vi "WriteClock.vi"(6 "Error In":errorcluster, 7 "Time & Date":u8[](array[numeric])=[0], 8 "Cluster":T1, 9 "LINX Resource":T2={"IO"=enum."Remote", "Interface"=enum."Serial", "LINX Device Config"={"Interface"=enum."Serial", "COM Port"="COM13", "TCP Configuration"={"IP Address"="", "Port"=0}, "Device Family"=1, "Device ID"=1, "Device Name"="myRIO-1900", "TCP Ref"=refnum, "Channels"={"DI"=[0, 1, 2, 3, 4, 5, 6, 7, 8, 9, 10, 11, 12, 13, 14, 15, 16, 17, 18, 19, 20, 21, 22, 23, 24, 25, 26, 27, 28, 29, 30, 31, 32, 33, 34, 35, 36, 37, 38, 39, 40, 41, 42, 43, 44, 45, 46], "DO"=[0, 1, 2, 3, 4, 5, 6, 7, 8, 9, 10, 11, 12, 13, 14, 15, 16, 17, 18, 19, 20, 21, 22, 23, 24, 25, 26, 27, 28, 29, 30, 31, 32, 33, 34, 35, 36, 37, 38, 39, 40, 41, 42, 43, 44, 45, 46], "AI"=[0, 1, 2, 3, 4, 5, 6, 7, 8, 9, 10, 11], "AO"=[], "PWM"=[3, 5, 6, 9, 10], "QE"=[], "UART"=[0, 1], "I2C 2"=[0], "SPI"=[0], "CAN"=[], "Servo"=[], "AI Ref (V)"=0.0, "AI Resolution (Bits)"=0, "AO Ref (V)"=0.0, "AO Resolution (Bits)"=0}}}) -> (0 "Error Out":errorcluster, 3 "LINX Resource":T2={"IO"=enum."Remote", "Interface"=enum."Serial", "LINX Device Config"={"Interface"=enum."Serial", "COM Port"="COM13", "TCP Configuration"={"IP Address"="", "Port"=0}, "Device Family"=1, "Device ID"=1, "Device Name"="myRIO-1900", "TCP Ref"=refnum, "Channels"={"DI"=[0, 1, 2, 3, 4, 5, 6, 7, 8, 9, 10, 11, 12, 13, 14, 15, 16, 17, 18, 19, 20, 21, 22, 23, 24, 25, 26, 27, 28, 29, 30, 31, 32, 33, 34, 35, 36, 37, 38, 39, 40, 41, 42, 43, 44, 45, 46], "DO"=[0, 1, 2, 3, 4, 5, 6, 7, 8, 9, 10, 11, 12, 13, 14, 15, 16, 17, 18, 19, 20, 21, 22, 23, 24, 25, 26, 27, 28, 29, 30, 31, 32, 33, 34, 35, 36, 37, 38, 39, 40, 41, 42, 43, 44, 45, 46], "AI"=[0, 1, 2, 3, 4, 5, 6, 7, 8, 9, 10, 11], "AO"=[], "PWM"=[3, 5, 6, 9, 10], "QE"=[], "UART"=[0, 1], "I2C 2"=[0], "SPI"=[0], "CAN"=[], "Servo"=[], "AI Ref (V)"=0.0, "AI Resolution (Bits)"=0, "AO Ref (V)"=0.0, "AO Resolution (Bits)"=0}}})   [LabVIEW 2024]
uses:
  <vilib>/MakerHub/LINX/Private/Type Defs/LINX Ref.ctl
  <vilib>/MakerHub/LINX/Private/Type Defs/Platform.ctl
  <vilib>/MakerHub/LINX/Private/Type Defs/Interface.ctl
  <vilib>/MakerHub/LINX/Private/Device/Type Defs/LINX Device Config.ctl
  <vilib>/MakerHub/LINX/Private/Device/Type Defs/TCP Config.ctl
  <vilib>/MakerHub/LINX/Private/Device/Type Defs/Channels.ctl
  <vilib>/MakerHub/LINX/Private/Local IO/LinxI2cWrite.vi
  <vilib>/MakerHub/LINX/Public/Utilities/Check Channel.vi
  <vilib>/MakerHub/LINX/Private/Local IO/Handle Errors.vi
  <vilib>/MakerHub/LINX/Private/Utilties/Generate Error.vi
  <vilib>/MakerHub/LINX/LMH-LINX.lvlib
  <vilib>/MakerHub/LINX/Private/Device/Device.lvlib
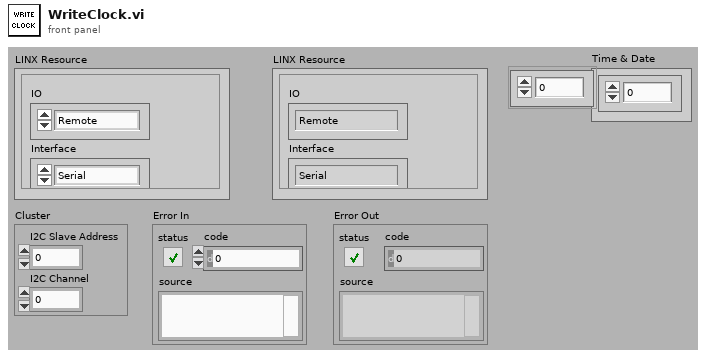
[diagram p1: front panel]
types:
  T1 = cluster{"I2C Slave Address":u8, "I2C Channel":u8}
  T2 = typedef "LMH-LINX.lvlib/LINX Ref.ctl" = cluster{"IO":T3, "Interface":T4, "LINX Device Config":T5}
  T3 = typedef "LMH-LINX.lvlib/Platform.ctl" = enum16{"Remote", "Local"}
  T4 = typedef "LMH-LINX.lvlib/Interface.ctl" = enum16{"Serial", "TCP"}
  T5 = typedef "LMH-LINX.lvlib/Device.lvlib/LINX Device Config.ctl" = cluster{"Interface":T4, "COM Port":refnum<visa-resource-name>, "TCP Configuration":T6, "Device Family":u8, "Device ID":u8, "Device Name":string, "TCP Ref":refnum<k5>, "Channels":T7}
  T6 = typedef "LMH-LINX.lvlib/Device.lvlib/TCP Config.ctl" = cluster{"IP Address":string, "Port":u16}
  T7 = typedef "LMH-LINX.lvlib/Channels.ctl" = cluster{"DI":u8[], "DO":u8[], "AI":u8[], "AO":u8[], "PWM":u8[], "QE":u8[], "UART":u8[], "I2C 2":u8[], "SPI":u8[], "CAN":u8[], "Servo":u8[], "AI Ref (V)":dbl, "AI Resolution (Bits)":u8, "AO Ref (V)":dbl, "AO Resolution (Bits)":u8}
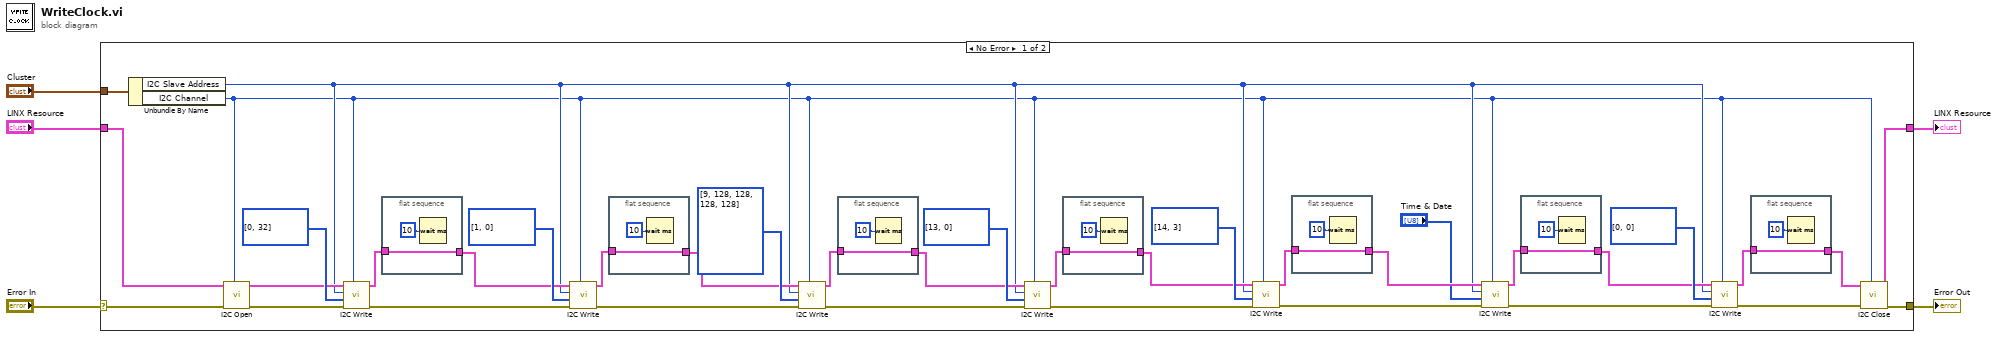
[diagram p0: block diagram]
diagram:
  n1 = case shown="No Error" "Error In" {
    selector: "Error In" -> [w35 w58]
    tunnel: [w41 w58] -> w3
    tunnel: "LINX Resource" -> [w42 w57]
    tunnel: [w40 w57] -> w4
    tunnel: "Cluster" -> [w34 _]
    frame No Error {
      n2 = Unbundle By Name(w34) -> ("I2C Slave Address"=w8:u8, "I2C Channel"=w7:u8)
      n3 = call <vilib>:"I2C Open.vi"("I2C Channel (0)"=w7, "Error In"=w35, "LINX Resource"=w42) -> ("Error Out"=w36:errorcluster, "LINX Resource"=w38:T2)  [unwired: 7 in]
      n4 = call <vilib>:"I2C Write.vi"("I2C Channel"=w7, "Error In"=w36, "Data"=u8[] [0, 32], "I2C Slave Address (0)"=w8, "LINX Resource"=w38) -> ("Error Out"=w26:errorcluster, "LINX Resource"=w37:T2)  [unwired: 5 in]
      n5 = flat-sequence {
        tunnel: [w56] -> w27
        tunnel: w37 -> [w56]
        frame #0 {
          n6 = Wait (ms)(milliseconds to wait=u32 10) -> ()  [unwired: 1 out]
        }
      }
      n7 = call <vilib>:"I2C Write.vi"("I2C Channel"=w7, "Error In"=w26, "Data"=u8[] [1, 0], "I2C Slave Address (0)"=w8, "LINX Resource"=w27) -> ("Error Out"=w25:errorcluster, "LINX Resource"=w33:T2)  [unwired: 5 in]
      n8 = flat-sequence {
        tunnel: [w54] -> w24
        tunnel: w33 -> [w54]
        frame #0 {
          n9 = Wait (ms)(milliseconds to wait=u32 10) -> ()  [unwired: 1 out]
        }
      }
      n10 = call <vilib>:"I2C Write.vi"("I2C Channel"=w7, "Error In"=w25, "Data"=u8[] [9, 128, 128, 128, 128], "I2C Slave Address (0)"=w8, "LINX Resource"=w24) -> ("Error Out"=w23:errorcluster, "LINX Resource"=w30:T2)  [unwired: 5 in]
      n11 = flat-sequence {
        tunnel: [w52] -> w22
        tunnel: w30 -> [w52]
        frame #0 {
          n12 = Wait (ms)(milliseconds to wait=u32 10) -> ()  [unwired: 1 out]
        }
      }
      n13 = call <vilib>:"I2C Write.vi"("I2C Channel"=w7, "Error In"=w23, "Data"=u8[] [13, 0], "I2C Slave Address (0)"=w8, "LINX Resource"=w22) -> ("Error Out"=w12:errorcluster, "LINX Resource"=w29:T2)  [unwired: 5 in]
      n14 = flat-sequence {
        tunnel: [w50] -> w16
        tunnel: w29 -> [w50]
        frame #0 {
          n15 = Wait (ms)(milliseconds to wait=u32 10) -> ()  [unwired: 1 out]
        }
      }
      n16 = call <vilib>:"I2C Write.vi"("I2C Channel"=w7, "Error In"=w12, "Data"=u8[] [14, 3], "I2C Slave Address (0)"=w8, "LINX Resource"=w16) -> ("Error Out"=w11:errorcluster, "LINX Resource"=w20:T2)  [unwired: 5 in]
      n17 = flat-sequence {
        tunnel: [w48] -> w15
        tunnel: w20 -> [w48]
        frame #0 {
          n18 = Wait (ms)(milliseconds to wait=u32 10) -> ()  [unwired: 1 out]
        }
      }
      n19 = call <vilib>:"I2C Write.vi"("I2C Channel"=w7, "Error In"=w11, "Data"="Time & Date", "I2C Slave Address (0)"=w8, "LINX Resource"=w15) -> ("Error Out"=w10:errorcluster, "LINX Resource"=w19:T2)  [unwired: 5 in]
      n20 = flat-sequence {
        tunnel: [w46] -> w14
        tunnel: w19 -> [w46]
        frame #0 {
          n21 = Wait (ms)(milliseconds to wait=u32 10) -> ()  [unwired: 1 out]
        }
      }
      n22 = call <vilib>:"I2C Write.vi"("I2C Channel"=w7, "Error In"=w10, "Data"=u8[] [0, 0], "I2C Slave Address (0)"=w8, "LINX Resource"=w14) -> ("Error Out"=w9:errorcluster, "LINX Resource"=w17:T2)  [unwired: 5 in]
      n23 = flat-sequence {
        tunnel: [w44] -> w13
        tunnel: w17 -> [w44]
        frame #0 {
          n24 = Wait (ms)(milliseconds to wait=u32 10) -> ()  [unwired: 1 out]
        }
      }
      n25 = call <vilib>:"I2C Close.vi"("I2C Channel (0)"=w7, "Error In"=w9, "LINX Resource"=w13) -> ("Error Out"=w41:errorcluster, "LINX Resource"=w40:T2)  [unwired: 7 in]
    }
    frame Error {
    }
  }
  "LINX Resource" <- w4
  "Error Out" <- w3
